vi "prepare child task.vi"(10 "child task in":refnum<class "task.lvclass">, 11 "task in":refnum<class "task.lvclass">) -> (2 "child task out":refnum<class "task.lvclass">, 3 "task out":refnum<class "task.lvclass">)   [LabVIEW 2013, in "task.lvclass"]
uses:
  task.lvclass
  task.lvclass/task.ctl
  dispatcher/thread pool.lvclass
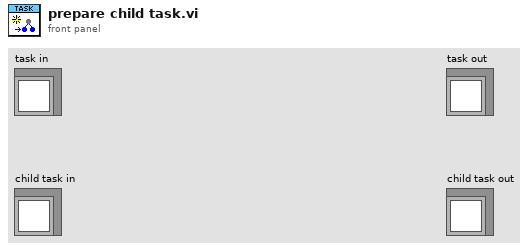
[diagram p1: front panel]
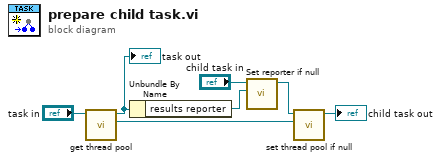
[diagram p0: block diagram]
diagram:
  n1 = call "get thread pool.vi"("task in"="task in") -> ("dispatcher"=w1:refnum<data-value>, "task out"=w2:refnum<class "task.lvclass">)  [unwired: 9 in]
  "task out" <- w2
  n2 = Unbundle By Name(w2) -> ("results reporter"=w4:refnum<class "results reporter.lvclass">)
  n3 = call "Set reporter if null.vi"("results reporter"=w4, "task in"="child task in") -> ("task out"=w7:refnum<class "task.lvclass">)  [unwired: 9 in]
  n4 = call "set thread pool if null.vi"("dispatcher"=w1, "task in"=w7) -> ("task out"=→"child task out":refnum<class "task.lvclass">)  [unwired: 9 in]
